vi "Write Device Description JSON.vi"(8 "error in (no error)":errorcluster, 10 "Device Description JSON":string, 11 "Control Experiment in":refnum<class "Control Experiment SM.lvclass">) -> (0 "error out":errorcluster, 3 "Control Experiment out":refnum<class "Control Experiment SM.lvclass">)   [LabVIEW 2016, in "Control Experiment SM.lvclass"]
uses:
  Control Experiment SM.lvclass
  Control Experiment SM.lvclass/Control Experiment SM.ctl
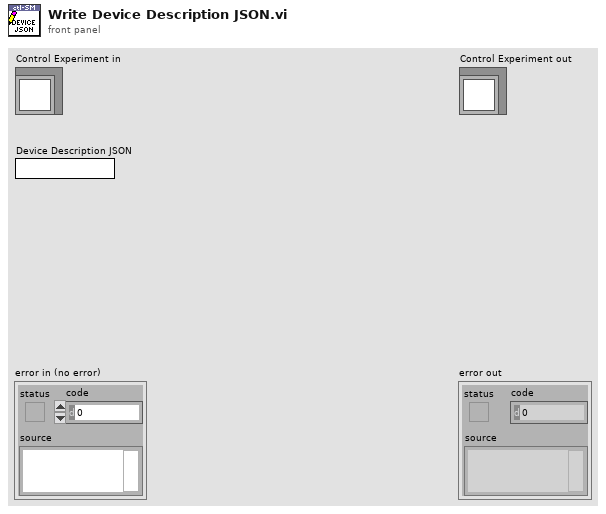
[diagram p1: front panel]
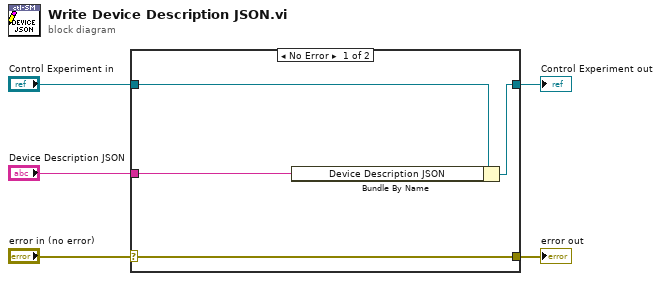
[diagram p0: block diagram]
diagram:
  n1 = case shown="No Error" "error in (no error)" {
    selector: "error in (no error)" -> [w9 w10]
    tunnel: [w9 w10] -> w4
    tunnel: [w7 w11] -> w2
    tunnel: "Control Experiment in" -> [w8 w11]
    tunnel: "Device Description JSON" -> [w6 _]
    frame No Error {
      n2 = Bundle By Name(cluster=w8, "Device Description JSON"=w6) -> (w7:refnum<class "Control Experiment SM.lvclass">)
    }
    frame Error {
    }
  }
  "error out" <- w4
  "Control Experiment out" <- w2
